vi "Str2HexStr.vi"(7 "data out":string) -> (8 "String":string)   [LabVIEW 2011]
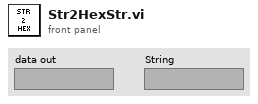
[diagram p1: front panel]
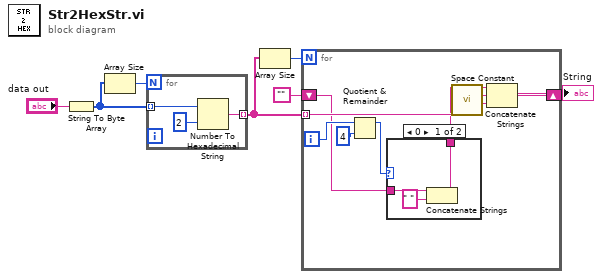
[diagram p0: block diagram]
diagram:
  n1 = String To Byte Array(string="data out") -> (unsigned byte array=w2:u8[])
  n2 = Array Size(array=w2) -> (size(s)=w3:i32)
  n3 = for {
    N: w3 -> [_]
    tunnel: w2 -> [w10] mode=indexing
    tunnel: [w8] -> w5 mode=indexing
    n4 = Number To Hexadecimal String(1:i16 2 ("width (-)"), 2:w10) -> (0:w8:string)
  }
  n5 = Array Size(array=w5) -> (size(s)=w4:i32)
  n6 = for {
    N: w4 -> [_]
    tunnel: w5 -> [w16] mode=indexing
    shift-right: [w18] -> w7
    shift-left: "" -> [w12]
    i -> [w15]
    n7 = Quotient & Remainder(x=w15, y=4) -> (x-y*floor(x/y)=w13:i32)  [unwired: 1 out]
    n8 = case shown="0" w13 {
      tunnel: w12 -> [w21 w22]
      tunnel: [w19 w22] -> w11
      frame 0 {
        n9 = Concatenate Strings(w21, " " ("string")) -> (w19:string)
      }
      frame 1, Default {
      }
    }
    n10 = call <vilib>:"Space Constant.vi"() -> ("String"=w17:string)
    n11 = Concatenate Strings(w11, w17, w16) -> (w18:string)
  }
  "String" <- w7
